vi "libssh2_sftp_stat.vi"(8 "error in (no error)":errorcluster, 10 "path":string, 11 "sftp":T2) -> (0 "error out":errorcluster, 2 "attributes":T1)   [LabVIEW 2013, in "libssh2.lvlib"]
doc: "Read information about the file referred to by path. If path is a symbolic link then the information about the file it refers to is returned."
uses:
  SFTP Refnum.ctl
  libssh2_sftp_attributes.ctl
  libssh2_sftp_stat_type.ctl
  libssh2.lvlib
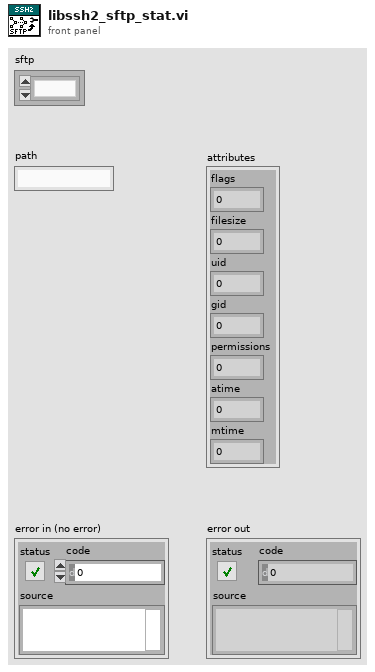
[diagram p1: front panel]
types:
  T1 = typedef "libssh2.lvlib/libssh2_sftp_attributes.ctl" = cluster{"flags":u32, "filesize":u64, "uid":u32, "gid":u32, "permissions":u32, "atime":u32, "mtime":u32}
  T2 = typedef "libssh2.lvlib/SFTP Refnum.ctl" = refnum<k1>
  T3 = typedef "libssh2.lvlib/libssh2_sftp_stat_type.ctl" = enum16{"STAT", "LSTAT", "SETSTAT"}
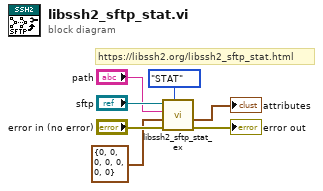
[diagram p0: block diagram]
diagram:
  # "https://libssh2.org/libssh2_sftp_stat.html"
  n1 = call "libssh2_sftp_stat_ex.vi"("stat type"=libssh2_sftp_stat_type."STAT", "error in (no error)"="error in (no error)", "attributes in"=T1 {"flags"=0, "filesize"=0, "uid"=0, "gid"=0, "permissions"=0, "atime"=0, "mtime"=0}, "path"="path", "sftp"="sftp") -> ("error out"=→"error out":errorcluster, "attributes out"=→"attributes":T1)  [unwired: 5 in]
